vi "Create WavBuf.vi"(5 "Scale Offset":cluster{"Slope":dbl, "Intercept":dbl}={"Slope"=1.0, "Intercept"=0.0} {"Intercept" format="%.6g"; "Slope" format="%.6g"}, 6 "Units":string, 7 "Name":string, 8 "Error":errorcluster, 9 "Samples/Sec":dbl, 10 "Buffer Size(S)":dbl, 11 "(WavBuf)":refnum<class "(WavBuf).lvclass">) -> (0 "Error Out":errorcluster, 3 "(WavBuf) Out":refnum<class "(WavBuf).lvclass">)   [LabVIEW 2016, in "(WavBuf).lvclass"]
uses:
  (WavBuf).lvclass
  Pointer/((Pointer)).lvclass
  Universal Controls/Read Write Button.ctl
  Universal Controls/Waveform_Data.ctl
  (WavBuf).lvclass/(WavBuf).ctl
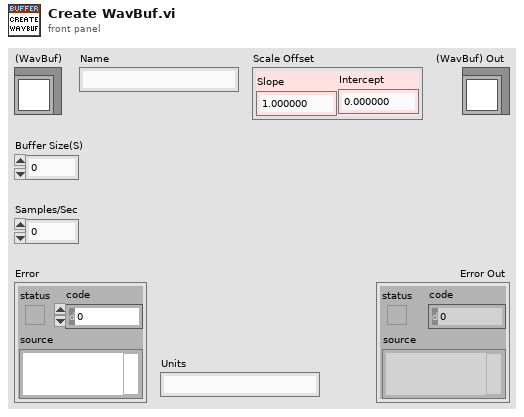
[diagram p1: front panel]
types:
  T1 = typedef "Waveform_Data.ctl" = waveform(dbl)
  T2 = typedef "Read Write Button.ctl" = bool
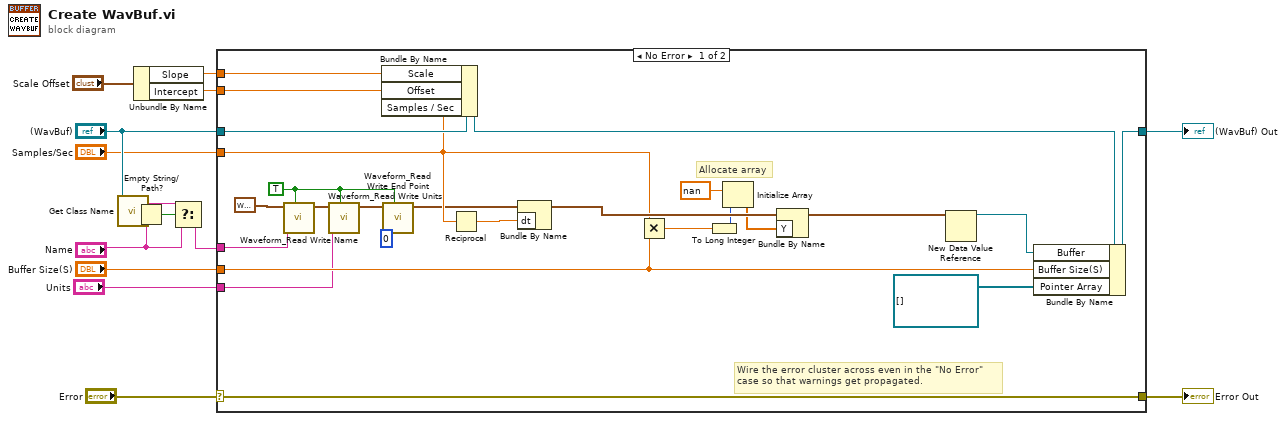
[diagram p0: block diagram]
diagram:
  n1 = call "Get Class Name.vi"("lvclass"="(WavBuf)") -> ("Child Name"=w9:string)  [unwired: 3 in, 1 out]
  n2 = Unbundle By Name("Scale Offset") -> ("Slope"=w3:dbl, "Intercept"=w2:dbl)
  n3 = Empty String/Path?(string/path="Name") -> (empty?=w10:bool)
  n4 = Select(t=w9, s=w10, f="Name") -> (s? t:f=w7:string)
  n5 = case shown="No Error" "Error" {
    selector: "Error" -> [w39 w41]
    tunnel: [w39 w41] -> w13
    tunnel: [w38 w40] -> w5
    tunnel: "(WavBuf)" -> [w29 w40]
    tunnel: "Buffer Size(S)" -> [w33 _]
    tunnel: w7 -> [w35 _]
    tunnel: "Samples/Sec" -> [w27 _]
    tunnel: w2 -> [w26 _]
    tunnel: w3 -> [w23 _]
    tunnel: "Units" -> [w16 _]
    frame No Error {
      w15 = T2 TRUE ("Read(f)\nWrite(t)")
      # "Allocate array"
      # "Wire the error cluster across even in the \"No Error\"\ncase so that warnings get propagated."
      n6 = call "Waveform_Read Write Name.vi"("Read(f)\nWrite(t)"=w15, "Name"=w35, "Raw Data Waveform"=T1 {"t0"=timestamp(0 s since 1904-01-01), "dt"=1.0, "Y"=[]}) -> ("Raw Data Waveform Out"=w18:T1)  [unwired: 7 in, 1 out]
      n7 = call "Waveform_Read Write Units.vi"("Read(f)\nWrite(t)"=w15, "Name"=w16, "Raw Data Waveform"=w18) -> ("Raw Data Waveform Out"=w17:T1)  [unwired: 7 in, 1 out]
      n8 = Bundle By Name(cluster=w29, "Scale"=w23, "Offset"=w26, "Samples / Sec"=w27) -> (w28:refnum<class "(WavBuf).lvclass">)
      n9 = call "Waveform_Read Write End Point.vi"("Read(f)\nWrite(t)"=w15, "End Point"=0, "Raw Data Waveform"=w17) -> ("Raw Data Waveform Out"=w25:T1)  [unwired: 7 in, 1 out]
      n10 = Reciprocal(x=w27) -> (1/x=w30:dbl)
      n11 = Bundle By Name(cluster=w25, "dt"=w30) -> (w31:T1)
      n12 = Multiply(x=w27, y=w33) -> (x*y=w19:dbl)
      n13 = To Long Integer(number=w19) -> (32bit integer=w20:i32)
      n14 = Initialize Array(nan ("Buffer Size(S)"), w20) -> (w21:dbl[])
      n15 = Bundle By Name(cluster=w31, "Y"=w21) -> (w34:T1)
      n16 = New Data Value Reference(data value=w34) -> (data value reference=w37:refnum<data-value>)  [unwired: 1 in, 1 out]
      n17 = Bundle By Name(cluster=w28, "Buffer"=w37, "Buffer Size(S)"=w33, "Pointer Array"=refnum<class "((Pointer)).lvclass">[] []) -> (w38:refnum<class "(WavBuf).lvclass">)
    }
    frame Error {
    }
  }
  "Error Out" <- w13
  "(WavBuf) Out" <- w5
